vi "Sequence file type text with dot.vi"() -> (8 "Sequrncefile type with dot":string, 10 "Sequrncefile type without dot":string)   [LabVIEW 2011]
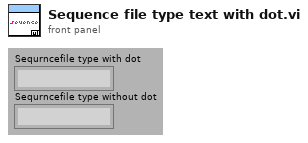
[diagram p1: front panel]
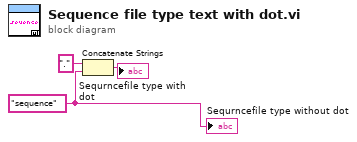
[diagram p0: block diagram]
diagram:
  w1 = "sequence" ("string")
  n1 = Concatenate Strings("." ("string"), w1) -> (→"Sequrncefile type with dot":string)
  "Sequrncefile type without dot" <- w1
